vi "Prueba_p_crear_ruta.vi"() -> ()   [LabVIEW 2019]
panel:
  out "path 2":path
  in  "path":path
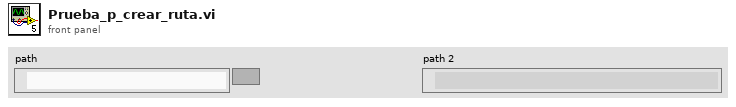
[diagram p1: front panel]
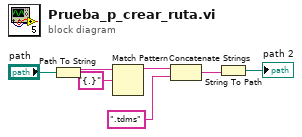
[diagram p0: block diagram]
diagram:
  n1 = Path To String(path="path") -> (string=w6:string)
  n2 = Match Pattern(string=w6, regular expression="{.}") -> (before substring=w4:string)  [unwired: 1 in, 3 out]
  n3 = Concatenate Strings(w4, ".tdms" ("string")) -> (w2:string)
  n4 = String To Path(string=w2) -> (path=→"path 2":path)
